vi "Class Object Construction.vi"(6 "class":T1=enum."Valve Controller", 7 "error in":errorcluster, 8 "param2":variant, 9 "param 1":variant, 10 "classes in":T2) -> (0 "error out":errorcluster, 3 "classes out":T2)   [LabVIEW 2011]
uses:
  Controls/Class Objects.ctl
  Modules/File/Configuration/Configuration.lvclass
  Modules/Hardware/Power Supply/Power Supply.lvclass
  Modules/Hardware/Mass Flow Controller/Mass Flow Controller.lvclass
  Modules/Hardware/PID/PID.lvclass
  Modules/Hardware/Valve Controller/Valve Controller.lvclass
  Modules/Hardware/Multimeter/Multimeter.lvclass
  Modules/Hardware/Vapour Generator/Vapour Generator.lvclass
  Modules/File/TDMS/TDMS.lvclass
  Controls/Class Labels.ctl
  Modules/File/Configuration/File Type.ctl
  Controls/TDMS File Handling.ctl
  Functional Global Data/Globals.ctl
  Functional Global Data/Device Params Global.ctl
  Modules/Hardware/INL PID/INL PID.lvclass
  Modules/Hardware/Baseline Mocon piD-Tech plus/Baseline Mocon piD-Tech plus.lvclass
  Modules/Hardware/Stanford Research PS350/Stanford Research PS350.lvclass
  Modules/Hardware/Keithley 2400/Keithley 2400.lvclass
  Modules/Hardware/Owlstone GEN-SYS/Owlstone GEN-SYS.lvclass
  Modules/Hardware/Aalborg GFC17/Aalborg GFC17.lvclass
  Modules/Hardware/INL Valve Controller/INL Valve Controller.lvclass
  Modules/Hardware/Agilent 3458A/Agilent 3458A.lvclass
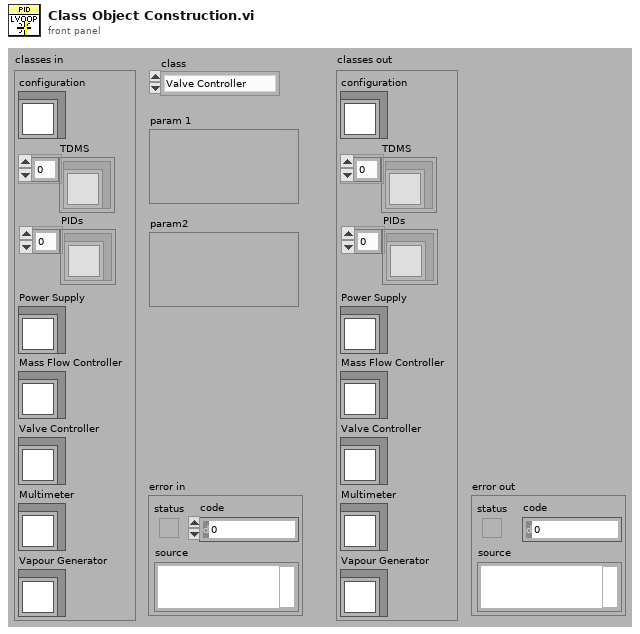
[diagram p1: front panel]
types:
  T1 = typedef "Class Labels.ctl" = enum16{"Configuration", "TDMS", "PID", "Power Supply", "Vapour Generator", "MFC", "NMR", "Valve Controller", "Multimeter"}
  T2 = typedef "Class Objects.ctl" = cluster{"configuration":refnum<class "Configuration.lvclass">, "TDMS":refnum<class "TDMS.lvclass">[], "Power Supply":refnum<class "Power Supply.lvclass">, "Mass Flow Controller":refnum<class "Mass Flow Controller.lvclass">, "Valve Controller":refnum<class "Valve Controller.lvclass">, "Multimeter":refnum<class "Multimeter.lvclass">, "Vapour Generator":refnum<class "Vapour Generator.lvclass">, "PIDs":refnum<class "PID.lvclass">[]}
  T3 = typedef "Configuration.lvclass/File Type.ctl" = enum16{"INI", "XML"}
  T4 = typedef "TDMS File Handling.ctl" = enum16{"Add TDMS File", "Get Active TDMS File", "Set Active TDMS File", "Set Active TDMS File Index"}
  T5 = typedef "Globals.ctl" = enum16{"Initialize", "Get DAQ Params", "Get Data Display Params", "Set DAQ Params", "Set Data Display Params"}
  T6 = typedef "Device Params Global.ctl" = enum16{"Initialize", "Get Device Settings", "Get Device Connections", "Set Device Settings", "Set Device Connections", "Get All Device Properties"}
  T7 = typedef "Data Acquisition Parameters.ctl" = cluster{"Experiment Type":T8, "Experiment Name":string, "Operator Name":string, "Notes":string, "TDMS File Path":path, "Data Acquisition State":bool, "PID Voltage Sweep":T9, "MFC Challenge Profile - Heaviside Step":T10, "MFC Challenge Profile":T11, "MFC Challenge Profile - Staircase":T12}
  T8 = typedef "DAQ Type.ctl" = enum16{"PID Sample", "PID with PS Challenge", "PID with MFC Challenge", "Multimeter Sample", "Multimeter with MFC Challenge"}
  T9 = typedef "PID Voltage Seep Settings.ctl" = cluster{"Voltage Step (V)":dbl, "Voltage Range (V)":cluster{u16, u16}, "Time Step (s)":dbl, "Voltage Step Direction":enum16{"High 2 Low", "Low 2 High"}}
  T10 = typedef "MFC Challenge Profile - Heaviside Step.ctl" = cluster{"Valve Open Duration":u16, "MFC Flow Rate":dbl, "Valve Open Repeats":u16, "Valve Open Start":u16}
  T11 = typedef "MFC Challen Profile Type.ctl" = enum16{"Heaviside", "Staircase"}
  T12 = typedef "MFC Challenge Profile - Staircase.ctl" = cluster{"Step Time Duration":u16, "Step Flow Rate":dbl, "Steps":u16, "Valve Open Start":u16, "Recovery":bool, "Repeats":u16}
  T13 = typedef "Device Connections.ctl" = cluster{"Detector":cluster{"Detector Type":T14, "Connection":bool, "B-M PID":T15, "INL PID Connections":T16}, "Power Supply":cluster{"Type":enum16{"Stanford Research PS350", "Keithley 2400"}, "Connection":bool, "VISA resource name":refnum<visa-resource-name>}, "Mass Flow Controller":cluster{"Type":enum16{"Aalborg GFC17"}, "Connection":bool, "Aalborg GFC17":T18}, "Valve Controller":cluster{"Type":T19, "Connection":bool, "SMC - INL":cluster{"VISA resource name":refnum<visa-resource-name>}}, "Multimeter":cluster{"Multimeter Type":T20, "Connection":bool, "VISA resource name":refnum<visa-resource-name>}, "Vapour Generator":cluster{"Type":T21, "Connection":bool, "Owlstone Gen-SYS":T22}}
  T14 = typedef "Detector Type.ctl" = enum16{"INL PID", "Baseline-Mocon piD-TECH plus"}
  T15 = typedef "Baseline Mocon piD-Tech plus.lvclass/Connections.ctl" = cluster{"AI DAQmx channel":tag}
  T16 = typedef "INL PID Connections.ctl" = cluster{"PIDs":u8, "Integrator DAQ Channels 1":T17, "Integrator DAQ Channels 2":T17}
  T17 = typedef "INL PID.lvclass/Integrator DAQmx Channels.ctl" = cluster{"V0":tag, "S1":tag, "S2":tag}
  T18 = typedef "Aalborg GFC17.lvclass/Aalborg GFC17 Connections.ctl" = cluster{"flow rate setpoint channel":tag, "flow rate reading channel":tag, "valve channel":tag}
  T19 = typedef "Valve Type.ctl" = enum16{"SMC - INL"}
  T20 = typedef "Multimeter Type.ctl" = enum16{"Agilent 3458A"}
  T21 = typedef "Vapour Generator Type.ctl" = enum16{"Owlstone GEN-SYS"}
  T22 = typedef "Owlstone GEN-SYS.lvclass/GEN-SYS Connections.ctl" = cluster{"GEN-SYS VISA resource name":refnum<visa-resource-name>, "OVG-4":cluster{"Flow Address":u8, "Temp Address":u8}, "OHG-4":cluster{"Flow Address":u8, "Easydew VISA resource name":refnum<visa-resource-name>}}
  T23 = enum16{"Stanford Research PS350", "Keithley 2400"}
  T24 = typedef "Device Settings.ctl" = cluster{"PID":cluster{"B-M PID":T25, "INL PID":T26}, "Power Supply":cluster{"Source Value":dbl, "Source Value Units":T27, "Source Mode":T28, "Limits":T29, "Output":bool}, "Mass Flow Controller":cluster{"MFC Flow Rate":dbl, "MFC Valve Status":T32}, "Valve Controller":cluster{"Valve Assembly":T33}, "Multimeter":cluster{"Agilent 3458A":cluster{"Measurement Configuration":T35, "Measurement Integration":T36}}, "Vapour Generator":cluster{"Owlstone Permeation Tube":T37, "Owlstone GEN-SYS Setpoints":T39}}
  T25 = typedef "Baseline Mocon piD-Tech plus.lvclass/Settings.ctl" = cluster{"Detector Sampling Frequency":dbl}
  T26 = typedef "INL PID.lvclass/Settings.ctl" = cluster{"Sampling Frequency":dbl, "Integration Time":dbl, "Integration Periods":u8, "Grid Voltage":dbl}
  T27 = typedef "Power Supply.lvclass/Source Units.ctl" = enum16{"volts", "millivolts", "microvolts", "amps", "milliamps", "microamps", "nanoamps"}
  T28 = typedef "Power Supply.lvclass/Source Mode.ctl" = enum16{"Volts", "Current"}
  T29 = typedef "Power Supply.lvclass/Protection Limits.ctl" = cluster{"Voltage Limit":dbl, "Voltage Limit Units":T30, "Current Limit":dbl, "Current Limit Units":T31, "Voltage Trip/Cmpl":dbl, "Voltage Trip/Cmpl Units":T30, "Current Trip/Cmpl":dbl, "Current Trip/Cmpl Units":T31}
  T30 = typedef "Power Supply.lvclass/Voltage Units.ctl" = enum16{"volts", "millivolts", "microvolts"}
  T31 = typedef "Power Supply.lvclass/Current Units.ctl" = enum16{"amps", "milliamps", "microamps", "nanoamps"}
  T32 = typedef "Mass Flow Controller.lvclass/Valve Status.ctl" = enum16{"Open", "Closed"}
  T33 = typedef "Valve Controller.lvclass/Valve Assembly.ctl" = cluster{"Valve 1":T34, "Valve 2":T34, "Valve 3":T34, "Valve 4":T34, "Valve 5":T34}
  T34 = typedef "Valve Controller.lvclass/Status.ctl" = u16
  T35 = typedef "Agilent 3458A.lvclass/Measurement Configuration.ctl" = cluster{"Function":enum16{"DC Voltage", "AC Voltage", "AC + DC Voltage", "DC Current", "AC Current", "AC + DC Current", "2-Wire Resistance", "4-Wire Resistance", "Frequency", "Period", "Direct Sampling DC", "Direct Sampling AC", "Sub-Sampling DC", "Sub-Sampling AC"}, " Manual Resolution":enum16{"4.5", "5.5", "6.5", "7.5", "8.5"}, "Frequency Source":enum16{"AC + DC Current", "AC + DC Voltage", "AC Current", "AC Voltage"}, "Auto Range":enum16{"OFF", "ON", "ONCE"}}
  T36 = typedef "Agilent 3458A.lvclass/Measurement Integration.ctl" = cluster{"Power Line Cycles":dbl}
  T37 = typedef "Owlstone GEN-SYS.lvclass/Permeation Tube.ctl" = cluster{"Tube":T38, "Molecular Weight":dbl, "Calibration Temperature\n(Celcius)":i32, "Permeation Rate \n(ng/min)":i32}
  T38 = typedef "Owlstone GEN-SYS.lvclass/Permeation Tube Gas.ctl" = enum16{"Isobutylene 27 Nov 2012", "Ammonia 29 Sep 2012", "DMMP Tube A 3 July 2014", "DMMP Tube B 3 July 2014"}
  T39 = typedef "Owlstone GEN-SYS.lvclass/Gen-Sys Setpoints.ctl" = cluster{"OVG-4":cluster{"Oven Temperature":i32, "Sample Flow Rate":i32, "Split Flow Status":u16, "Split Flow Rate":i32}, "OHG-4":cluster{"Wet Air Flow":i32}}
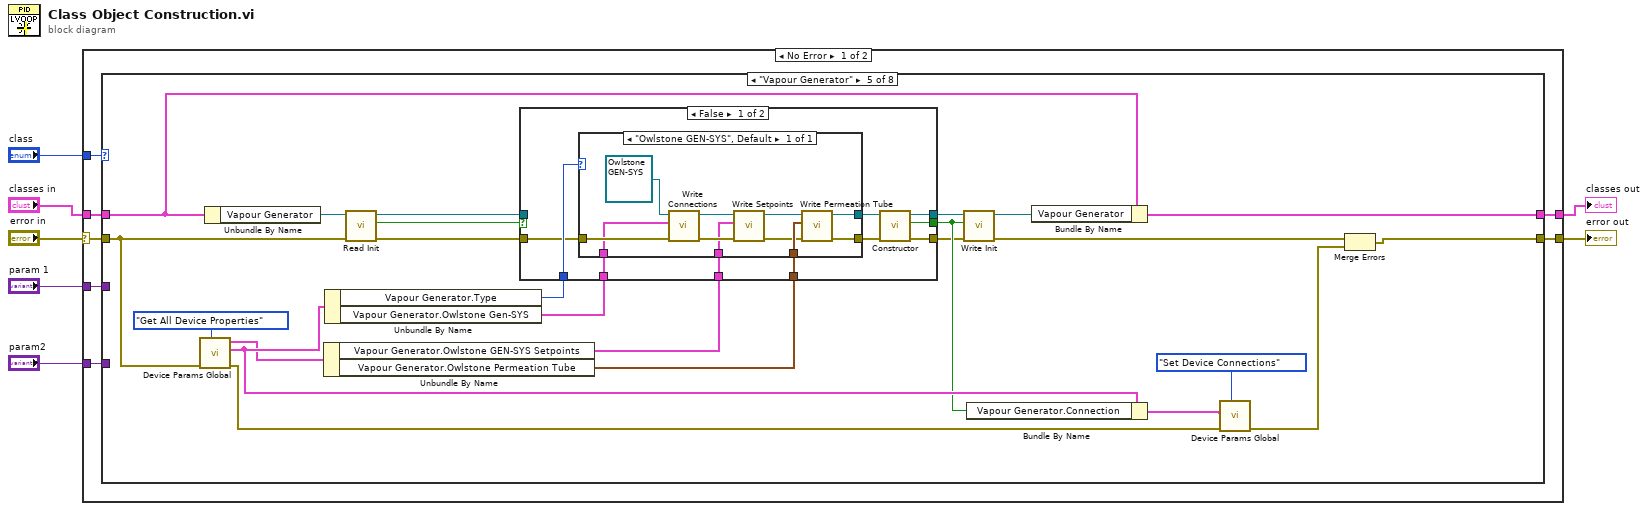
[diagram p0: block diagram]
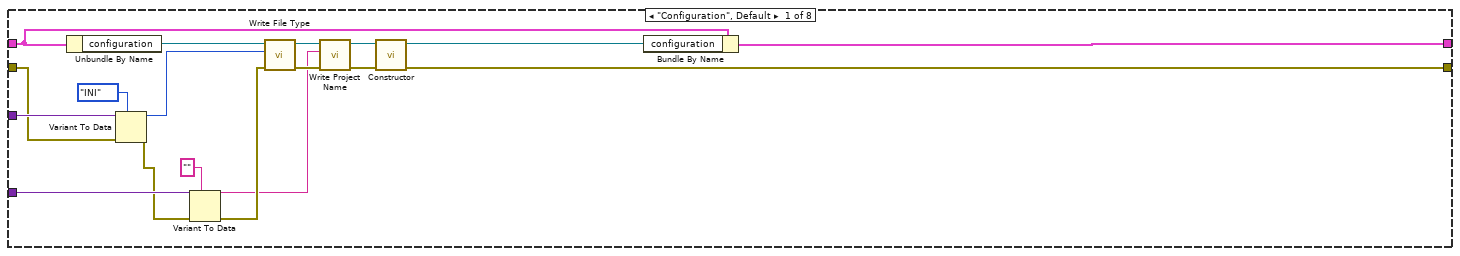
[diagram p2: hidden frame]
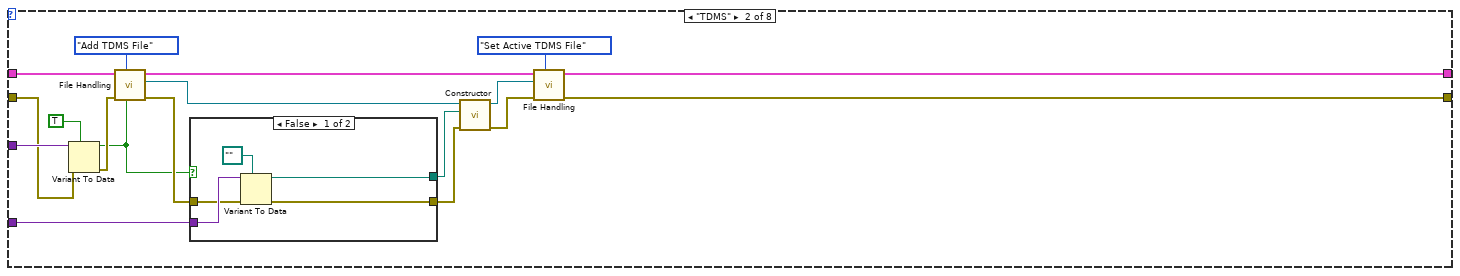
[diagram p3: hidden frame]
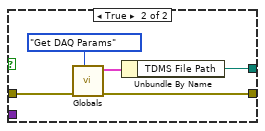
[diagram p4: hidden frame]
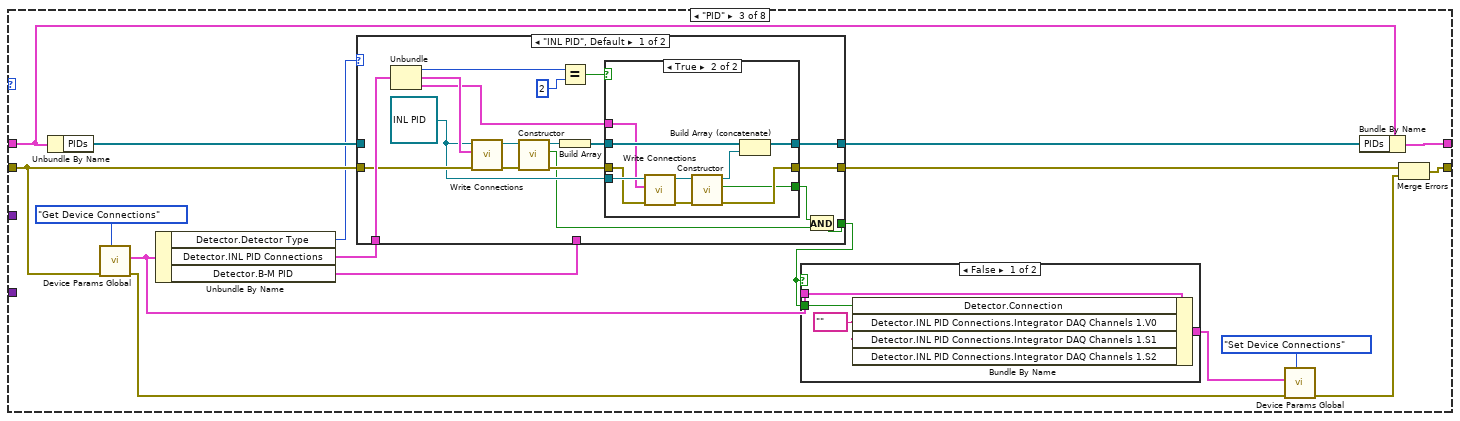
[diagram p5: hidden frame]
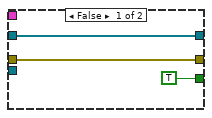
[diagram p6: hidden frame]
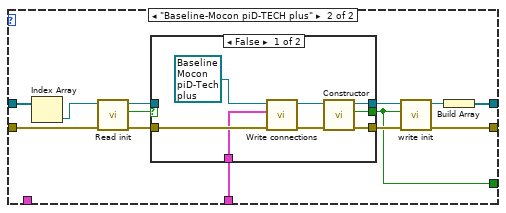
[diagram p7: hidden frame]
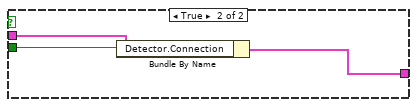
[diagram p9: hidden frame]
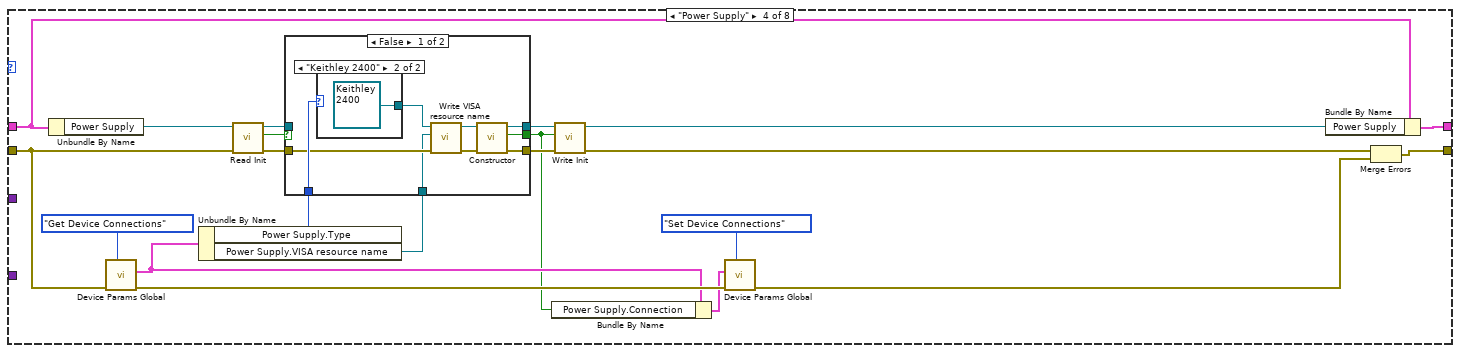
[diagram p10: hidden frame]
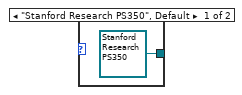
[diagram p11: hidden frame]
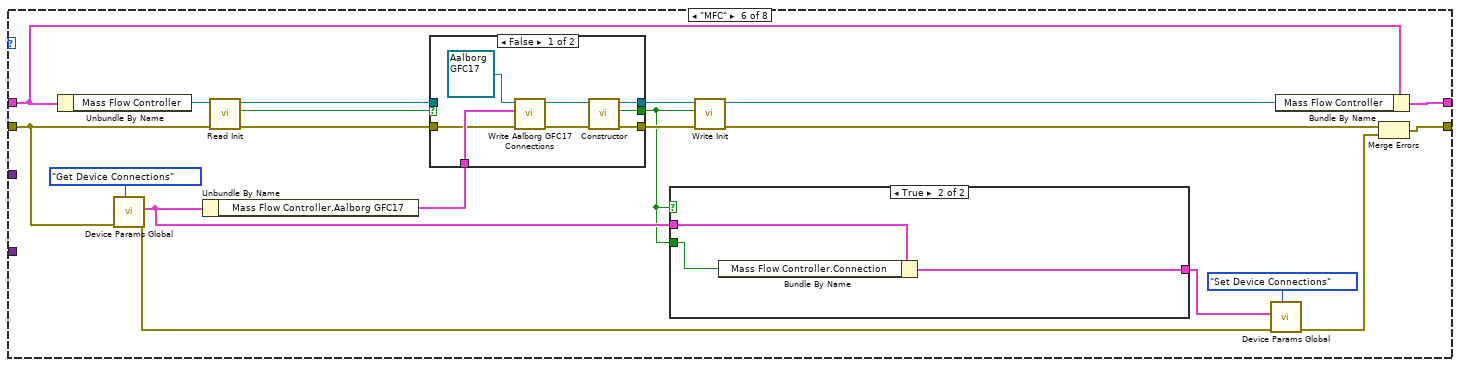
[diagram p14: hidden frame]
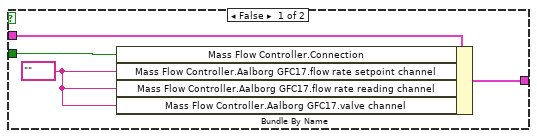
[diagram p15: hidden frame]
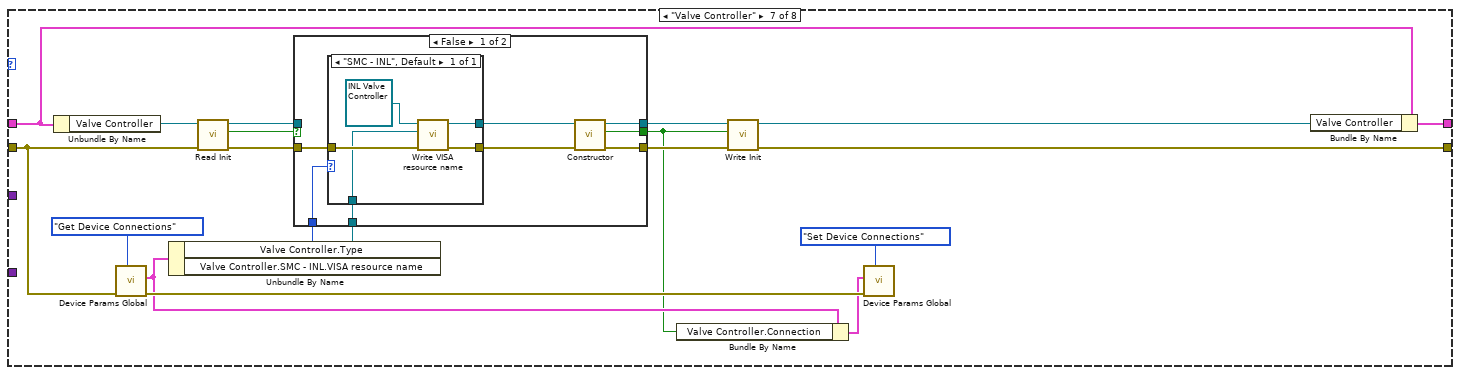
[diagram p17: hidden frame]
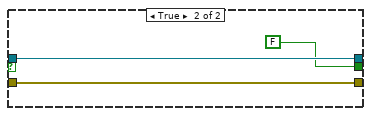
[diagram p18: hidden frame]
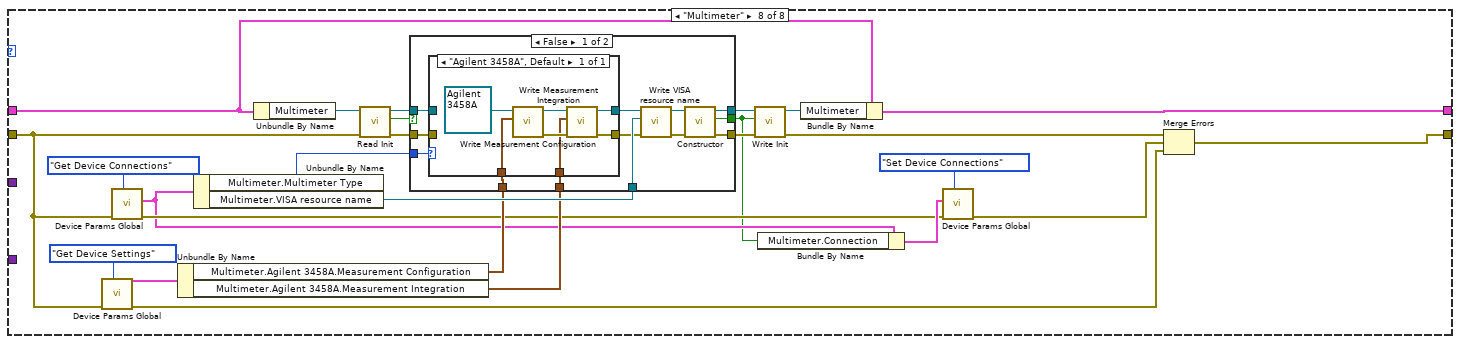
[diagram p19: hidden frame]
diagram:
  n1 = case shown="No Error" "error in" {
    selector: "error in" -> [w8 w346]
    tunnel: [w14 w346] -> w6
    tunnel: "classes in" -> [w13 w345]
    tunnel: "param 1" -> [w12 _]
    tunnel: "param2" -> [w11 _]
    tunnel: "class" -> [w10 _]
    tunnel: [w9 w345] -> w1
    frame No Error {
      n2 = case shown="\"Vapour Generator\"" w10 {
        tunnel: [w30 w43 w75 w154 w180 w229 w266 w310] -> w14
        tunnel: [w32 w44 w77 w156 w198 w237 w278 w320] -> w9
        tunnel: w13 -> [w27 w39 w76 w155 w187 w238 w279 w321]
        tunnel: w12 -> [w29 w40 _ _ _ _ _ _]
        tunnel: w11 -> [w20 w33 _ _ _ _ _ _]
        tunnel: w8 -> [w28 w38 w74 w152 w193 w235 w275 w307]
        frame "Configuration", Default {
          n3 = Unbundle By Name(w27) -> ("configuration"=w26:refnum<class "Configuration.lvclass">)
          n4 = Variant To Data(error in=w28, type=File_Type."INI" ("File Type"), Variant=w29) -> (data=w16:T3, error out=w19:errorcluster)
          n5 = Variant To Data(error in=w19, type="", Variant=w20) -> (data=w15:string, error out=w17:errorcluster)
          n6 = call-dynamic "Write File Type.vi"("error in (no error)"=w17, "File Type"=w16, "Configuration in"=w26) -> ("error out"=w22:errorcluster, "Configuration out"=w25:refnum<class "Configuration.lvclass">)  [unwired: 7 in]
          n7 = call-dynamic "Write Project Name.vi"("error in (no error)"=w22, "Project Name"=w15, "Configuration in"=w25) -> ("error out"=w23:errorcluster, "Configuration out"=w24:refnum<class "Configuration.lvclass">)  [unwired: 7 in]
          n8 = call-dynamic "Constructor.vi"("error in (no error)"=w23, "Configuration in"=w24) -> ("error out"=w30:errorcluster, "Configuration out"=w31:refnum<class "Configuration.lvclass">)  [unwired: 8 in]
          n9 = Bundle By Name(cluster=w27, "configuration"=w31) -> (w32:T2)
        }
        frame "TDMS" {
          n10 = Variant To Data(error in=w38, type=TRUE, Variant=w40) -> (data=w34:bool, error out=w48:errorcluster)
          n11 = call "File Handling.vi"("DAQ?"=w34, "TDMS File Handling"=TDMS_File_Handling."Add TDMS File", "error in"=w48, "Class objects"=w39) -> ("error out"=w37:errorcluster, "TDMS File"=w50:refnum<class "TDMS.lvclass">, "Class objects"=w47:T2)  [unwired: 5 in]
          n12 = case shown="False" w34 {
            tunnel: w37 -> [w53 w58]
            tunnel: [w51 w57] -> w36
            tunnel: [w52 w56] -> w35
            tunnel: w33 -> [w54 _]
            frame False {
              n13 = Variant To Data(error in=w53, type=path "", Variant=w54) -> (data=w52:path, error out=w51:errorcluster)
            }
            frame True {
              n14 = call "Globals.vi"("action"=Globals."Get DAQ Params", "error in"=w58) -> ("error out"=w57:errorcluster, "Data Acquisition"=w60:T7)  [unwired: 7 in, 1 out]
              n15 = Unbundle By Name(w60) -> ("TDMS File Path"=w56:path)
            }
          }
          n16 = call-dynamic "Constructor.vi"("error in"=w36, "path"=w35, "TDMS in"=w50) -> ("error out"=w42:errorcluster, "TDMS out"=w46:refnum<class "TDMS.lvclass">)  [unwired: 7 in]
          n17 = call "File Handling.vi"("TDMS File Handling"=TDMS_File_Handling."Set Active TDMS File", "error in"=w42, "TDMS File"=w46, "Class objects"=w47) -> ("error out"=w43:errorcluster, "Class objects"=w44:T2)  [unwired: 5 in, 1 out]
        }
        frame "PID" {
          n18 = Unbundle By Name(w76) -> ("PIDs"=w64:refnum<class "PID.lvclass">[])
          n19 = call "Device Params Global.vi"("action"=Device_Params_Global."Get Device Connections", "error in"=w74) -> ("error out"=w67:errorcluster, "Device Connections OUT"=w70:T13)  [unwired: 7 in, 1 out]
          n20 = Unbundle By Name(w70) -> ("Detector.Detector Type"=w63:T14, "Detector.INL PID Connections"=w71:T16, "Detector.B-M PID"=w65:T15)
          n21 = case shown="\"INL PID\", Default" w63 {
            tunnel: w74 -> [w92 w118]
            tunnel: [w81 w115] -> w72
            tunnel: w71 -> [w95 _]
            tunnel: w65 -> [_ w114]
            tunnel: w64 -> [_ w110]
            tunnel: [w82 w112] -> w62
            tunnel: [w78 w111] -> w61
            frame "INL PID", Default {
              w85 = refnum<class "INL PID.lvclass"> refnum ("PID.lvclass")
              n22 = Unbundle(w95) -> ("PIDs"=w89:u8, "Integrator DAQ Channels 1"=w94:T17, "Integrator DAQ Channels 2"=w84:T17)
              n23 = call-dynamic "Write Connections.vi"("error in (no error)"=w92, "Integrator DAQ Channels"=w94, "PID in"=w85) -> ("error out"=w91:errorcluster, "PID out"=w93:refnum<class "INL PID.lvclass">)  [unwired: 7 in]
              n24 = call-dynamic "Constructor.vi"("error in"=w91, "PID Detector in"=w93) -> ("error out"=w83:errorcluster, "init"=w80:bool, "PID Detector out"=w90:refnum<class "INL PID.lvclass">)  [unwired: 7 in]
              n25 = Equal?(x=w89, y=u8 2) -> (x = y?=w87:bool)
              n26 = Build Array(w90) -> (w86:refnum<class "INL PID.lvclass">[])
              n27 = case shown="True" w87 {
                tunnel: w86 -> [w98 w105]
                tunnel: w85 -> [_ w106]
                tunnel: w84 -> [_ w103]
                tunnel: w83 -> [w97 w102]
                tunnel: [w98 w101] -> w82
                tunnel: [w97 w100] -> w81
                tunnel: [TRUE ("init") w99] -> w79
                frame False {
                }
                frame True {
                  n28 = call-dynamic "Write Connections.vi"("error in (no error)"=w102, "Integrator DAQ Channels"=w103, "PID in"=w106) -> ("error out"=w107:errorcluster, "PID out"=w108:refnum<class "INL PID.lvclass">)  [unwired: 7 in]
                  n29 = call-dynamic "Constructor.vi"("error in"=w107, "PID Detector in"=w108) -> ("error out"=w100:errorcluster, "init"=w99:bool, "PID Detector out"=w104:refnum<class "INL PID.lvclass">)  [unwired: 7 in]
                  n30 = Build Array (concatenate)(w105, w104) -> (w101:refnum<class "INL PID.lvclass">[])
                }
              }
              n31 = And(x=w79, y=w80) -> (x .and. y?=w78:bool)
            }
            frame "Baseline-Mocon piD-TECH plus" {
              n32 = Index Array(array=w110) -> (element=w109:refnum<class "PID.lvclass">)  [unwired: 1 in]
              n33 = call-dynamic "Read init.vi"("error in (no error)"=w118, "Detector in"=w109) -> ("error out"=w119:errorcluster, "init"=w121:bool, "Detector out"=w120:refnum<class "PID.lvclass">)  [unwired: 7 in]
              n34 = case shown="False" w121 {
                selector: w121 -> [_ w130]
                tunnel: [w129 w132] -> w117
                tunnel: [w128 w131] -> w116
                tunnel: w120 -> [_ w132]
                tunnel: w119 -> [w127 w131]
                tunnel: [w124 w130] -> w111
                tunnel: w114 -> [w123 _]
                frame False {
                  n35 = call-dynamic "Write connections.vi"("error in (no error)"=w127, "Baseline-Mocon piD-TECH plus"=w123, "Baseline Mocon piD-Tech plus in"=refnum<class "Baseline Mocon piD-Tech plus.lvclass"> refnum ("Baseline Mocon piD-Tech plus.lvclass")) -> ("error out"=w125:errorcluster, "Baseline Mocon piD-Tech plus out"=w126:refnum<class "Baseline Mocon piD-Tech plus.lvclass">)  [unwired: 7 in]
                  n36 = call-dynamic "Constructor.vi"("error in"=w125, "Baseline Mocon \npiD-Tech plus in"=w126) -> ("error out"=w128:errorcluster, "init"=w124:bool, "Baseline Mocon \npiD-Tech plus out"=w129:refnum<class "Baseline Mocon piD-Tech plus.lvclass">)  [unwired: 7 in]
                }
                frame True {
                }
              }
              n37 = call-dynamic "write init.vi"("error in (no error)"=w116, "init?"=w111, "Detector in"=w117) -> ("error out"=w115:errorcluster, "Detector out"=w113:refnum<class "PID.lvclass">)  [unwired: 7 in]
              n38 = Build Array(w113) -> (w112:refnum<class "PID.lvclass">[])
            }
          }
          n39 = case shown="False" w61 {
            tunnel: w70 -> [w136 w139]
            tunnel: w61 -> [w135 w138]
            tunnel: [w133 w137] -> w68
            frame False {
              w134 = tag "" ("Detector.PID Connections.Integrator DAQ Channels.V0")
              n40 = Bundle By Name(cluster=w136, "Detector.Connection"=w135, "Detector.INL PID Connections.Integrator DAQ Channels 1.V0"=w134, "Detector.INL PID Connections.Integrator DAQ Channels 1.S1"=w134, "Detector.INL PID Connections.Integrator DAQ Channels 1.S2"=w134) -> (w133:T13)
            }
            frame True {
              n41 = Bundle By Name(cluster=w139, "Detector.Connection"=w138) -> (w137:T13)
            }
          }
          n42 = call "Device Params Global.vi"("action"=Device_Params_Global."Set Device Connections", "error in"=w67, "Device Connections IN"=w68) -> ("error out"=w66:errorcluster)  [unwired: 6 in, 2 out]
          n43 = Bundle By Name(cluster=w76, "PIDs"=w62) -> (w77:T2)
          n44 = Merge Errors(w72, w66) -> (w75:errorcluster)
        }
        frame "Power Supply" {
          n45 = Unbundle By Name(w155) -> ("Power Supply"=w160:refnum<class "Power Supply.lvclass">)
          n46 = call "Device Params Global.vi"("action"=Device_Params_Global."Get Device Connections", "error in"=w152) -> ("error out"=w144:errorcluster, "Device Connections OUT"=w143:T13)  [unwired: 7 in, 1 out]
          n47 = Unbundle By Name(w143) -> ("Power Supply.Type"=w151:T23, "Power Supply.VISA resource name"=w150:refnum<visa-resource-name>)
          n48 = call-dynamic "Read Init.vi"("error in (no error)"=w152, "Power Supply in"=w160) -> ("error out"=w158:errorcluster, "Init"=w159:bool, "Power Supply out"=w157:refnum<class "Power Supply.lvclass">)  [unwired: 7 in]
          n49 = case shown="False" w159 {
            selector: w159 -> [_ w172]
            tunnel: w158 -> [w165 w174]
            tunnel: w157 -> [_ w173]
            tunnel: [w167 w174] -> w147
            tunnel: [w168 w173] -> w149
            tunnel: w151 -> [w169 _]
            tunnel: [w166 w172] -> w142
            tunnel: w150 -> [w162 _]
            frame False {
              n50 = case shown="\"Keithley 2400\"" w169 {
                tunnel: [refnum<class "Stanford Research PS350.lvclass"> refnum ("Stanford Research PS350.lvclass") refnum<class "Keithley 2400.lvclass"> refnum ("Keithley 2400.lvclass")] -> w163
                frame "Stanford Research PS350", Default {
                }
                frame "Keithley 2400" {
                }
              }
              n51 = call-dynamic "Write VISA resource name.vi"("error in (no error)"=w165, "VISA resource name"=w162, "Power Supply in"=w163) -> ("error out"=w164:errorcluster, "Power Supply out"=w161:refnum<class "Power Supply.lvclass">)  [unwired: 7 in]
              n52 = call-dynamic "Constructor.vi"("error in (no error)"=w164, "Power Supply in"=w161) -> ("error out"=w167:errorcluster, "Init"=w166:bool, "Power Supply out"=w168:refnum<class "Power Supply.lvclass">)  [unwired: 7 in]
            }
            frame True {
            }
          }
          n53 = Bundle By Name(cluster=w143, "Power Supply.Connection"=w142) -> (w141:T13)
          n54 = call-dynamic "Write Init.vi"("error in (no error)"=w147, "Init"=w142, "Power Supply in"=w149) -> ("error out"=w146:errorcluster, "Power Supply out"=w148:refnum<class "Power Supply.lvclass">)  [unwired: 7 in]
          n55 = call "Device Params Global.vi"("action"=Device_Params_Global."Set Device Connections", "error in"=w144, "Device Connections IN"=w141) -> ("error out"=w140:errorcluster)  [unwired: 6 in, 2 out]
          n56 = Bundle By Name(cluster=w155, "Power Supply"=w148) -> (w156:T2)
          n57 = Merge Errors(w146, w140) -> (w154:errorcluster)
        }
        frame "Vapour Generator" {
          n58 = call "Device Params Global.vi"("action"=Device_Params_Global."Get All Device Properties", "error in"=w193) -> ("error out"=w176:errorcluster, "Device Connections OUT"=w195:T13, "Device Settings OUT"=w177:T24)  [unwired: 7 in]
          n59 = Unbundle By Name(w187) -> ("Vapour Generator"=w192:refnum<class "Vapour Generator.lvclass">)
          n60 = Unbundle By Name(w177) -> ("Vapour Generator.Owlstone GEN-SYS Setpoints"=w175:T39, "Vapour Generator.Owlstone Permeation Tube"=w178:T37)
          n61 = Unbundle By Name(w195) -> ("Vapour Generator.Type"=w188:T21, "Vapour Generator.Owlstone Gen-SYS"=w179:T22)
          n62 = call-dynamic "Read Init.vi"("error in (no error)"=w193, "Vapour Generator in"=w192) -> ("error out"=w190:errorcluster, "Init"=w191:bool, "Vapour Generator out"=w189:refnum<class "Vapour Generator.lvclass">)  [unwired: 7 in]
          n63 = case shown="False" w191 {
            selector: w191 -> [_ w220]
            tunnel: w190 -> [w207 w221]
            tunnel: w189 -> [_ w222]
            tunnel: w188 -> [w208 _]
            tunnel: [w204 w222] -> w186
            tunnel: [w203 w221] -> w184
            tunnel: [w202 w220] -> w185
            tunnel: w179 -> [w201 _]
            tunnel: w178 -> [w200 _]
            tunnel: w175 -> [w199 _]
            frame False {
              n64 = case shown="\"Owlstone GEN-SYS\", Default" w208 {
                tunnel: w207 -> [w219]
                tunnel: [w215] -> w206
                tunnel: [w216] -> w205
                tunnel: w201 -> [w217]
                tunnel: w200 -> [w214]
                tunnel: w199 -> [w209]
                frame "Owlstone GEN-SYS", Default {
                  n65 = call-dynamic "Write Connections.vi"("error in (no error)"=w219, "Connections"=w217, "Owlstone OVG-4 in"=refnum<class "Owlstone GEN-SYS.lvclass"> refnum ("Owlstone OVG-4.lvclass")) -> ("error out"=w213:errorcluster, "Owlstone OVG-4 out"=w211:refnum<class "Owlstone GEN-SYS.lvclass">)  [unwired: 7 in]
                  n66 = call-dynamic "Write Setpoints.vi"("error in (no error)"=w213, "Setpoints"=w209, "Owlstone GEN-SYS in"=w211) -> ("error out"=w212:errorcluster, "Owlstone GEN-SYS out"=w210:refnum<class "Owlstone GEN-SYS.lvclass">)  [unwired: 7 in]
                  n67 = call-dynamic "Write Permeation Tube.vi"("error in (no error)"=w212, "Permeation Tube"=w214, "Owlstone GEN-SYS in"=w210) -> ("error out"=w216:errorcluster, "Owlstone GEN-SYS out"=w215:refnum<class "Owlstone GEN-SYS.lvclass">)  [unwired: 7 in]
                }
              }
              n68 = call-dynamic "Constructor.vi"("error in"=w205, "Owlstone Gen-SYS in"=w206) -> ("error out"=w203:errorcluster, "Init"=w202:bool, "Owlstone GEN-SYS out"=w204:refnum<class "Owlstone GEN-SYS.lvclass">)  [unwired: 7 in]
            }
            frame True {
            }
          }
          n69 = call-dynamic "Write Init.vi"("error in (no error)"=w184, "Init"=w185, "Vapour Generator in"=w186) -> ("error out"=w182:errorcluster, "Vapour Generator out"=w183:refnum<class "Vapour Generator.lvclass">)  [unwired: 7 in]
          n70 = Bundle By Name(cluster=w195, "Vapour Generator.Connection"=w185) -> (w194:T13)
          n71 = Bundle By Name(cluster=w187, "Vapour Generator"=w183) -> (w198:T2)
          n72 = call "Device Params Global.vi"("action"=Device_Params_Global."Set Device Connections", "error in"=w176, "Device Connections IN"=w194) -> ("error out"=w181:errorcluster)  [unwired: 6 in, 2 out]
          n73 = Merge Errors(w182, w181) -> (w180:errorcluster)
        }
        frame "MFC" {
          n74 = Unbundle By Name(w238) -> ("Mass Flow Controller"=w242:refnum<class "Mass Flow Controller.lvclass">)
          n75 = call "Device Params Global.vi"("action"=Device_Params_Global."Get Device Connections", "error in"=w235) -> ("error out"=w225:errorcluster, "Device Connections OUT"=w228:T13)  [unwired: 7 in, 1 out]
          n76 = Unbundle By Name(w228) -> ("Mass Flow Controller.Aalborg GFC17"=w231:T18)
          n77 = call-dynamic "Read Init.vi"("error in (no error)"=w235, "Mass Flow Controller in"=w242) -> ("error out"=w240:errorcluster, "Init"=w241:bool, "Mass Flow Controller out"=w239:refnum<class "Mass Flow Controller.lvclass">)  [unwired: 7 in]
          n78 = case shown="False" w241 {
            selector: w241 -> [_ w258]
            tunnel: w240 -> [w250 w259]
            tunnel: [w256 w260] -> w233
            tunnel: [w255 w259] -> w234
            tunnel: w239 -> [_ w260]
            tunnel: [w257 w258] -> w227
            tunnel: w231 -> [w252 _]
            frame False {
              n79 = call-dynamic "Write Aalborg GFC17 Connections.vi"("error in (no error)"=w250, "Aalborg GFC17 Connections"=w252, "Aalborg GFC17 in"=refnum<class "Aalborg GFC17.lvclass"> refnum ("Aalborg GFC17.lvclass")) -> ("error out"=w254:errorcluster, "Aalborg GFC17 out"=w253:refnum<class "Aalborg GFC17.lvclass">)  [unwired: 7 in]
              n80 = call-dynamic "Constructor.vi"("error in (no error)"=w254, "Aalborg GFC17 in"=w253) -> ("error out"=w255:errorcluster, "Init"=w257:bool, "Aalborg GFC17 out"=w256:refnum<class "Aalborg GFC17.lvclass">)  [unwired: 7 in]
            }
            frame True {
            }
          }
          n81 = case shown="True" w227 {
            tunnel: w228 -> [w246 w249]
            tunnel: w227 -> [w245 w248]
            tunnel: [w243 w247] -> w226
            frame False {
              w244 = tag "" ("Mass Flow Controller.Aalborg GFC17 Connections.flow rate setpoint channel")
              n82 = Bundle By Name(cluster=w246, "Mass Flow Controller.Connection"=w245, "Mass Flow Controller.Aalborg GFC17.flow rate setpoint channel"=w244, "Mass Flow Controller.Aalborg GFC17.flow rate reading channel"=w244, "Mass Flow Controller.Aalborg GFC17.valve channel"=w244) -> (w243:T13)
            }
            frame True {
              n83 = Bundle By Name(cluster=w249, "Mass Flow Controller.Connection"=w248) -> (w247:T13)
            }
          }
          n84 = call-dynamic "Write Init.vi"("error in (no error)"=w234, "Init"=w227, "Mass Flow Controller in"=w233) -> ("error out"=w230:errorcluster, "Mass Flow Controller out"=w232:refnum<class "Mass Flow Controller.lvclass">)  [unwired: 7 in]
          n85 = call "Device Params Global.vi"("action"=Device_Params_Global."Set Device Connections", "error in"=w225, "Device Connections IN"=w226) -> ("error out"=w223:errorcluster)  [unwired: 6 in, 2 out]
          n86 = Bundle By Name(cluster=w238, "Mass Flow Controller"=w232) -> (w237:T2)
          n87 = Merge Errors(w230, w223) -> (w229:errorcluster)
        }
        frame "Valve Controller" {
          n88 = Unbundle By Name(w279) -> ("Valve Controller"=w276:refnum<class "Valve Controller.lvclass">)
          n89 = call "Device Params Global.vi"("action"=Device_Params_Global."Get Device Connections", "error in"=w275) -> ("error out"=w264:errorcluster, "Device Connections OUT"=w263:T13)  [unwired: 7 in, 1 out]
          n90 = Unbundle By Name(w263) -> ("Valve Controller.Type"=w271:T19, "Valve Controller.SMC - INL.VISA resource name"=w270:refnum<visa-resource-name>)
          n91 = call-dynamic "Read Init.vi"("error in (no error)"=w275, "Valve Controller in"=w276) -> ("error out"=w272:errorcluster, "Init"=w274:bool, "Valve Controller out"=w273:refnum<class "Valve Controller.lvclass">)  [unwired: 7 in]
          n92 = case shown="False" w274 {
            tunnel: [w287 w294] -> w268
            tunnel: [w286 w295] -> w269
            tunnel: w273 -> [_ w295]
            tunnel: w272 -> [w284 w294]
            tunnel: w271 -> [w285 _]
            tunnel: w270 -> [w283 _]
            tunnel: [w280 FALSE ("Init")] -> w262
            frame False {
              n93 = case shown="\"SMC - INL\", Default" w285 {
                tunnel: w284 -> [w292]
                tunnel: w283 -> [w291]
                tunnel: [w289] -> w282
                tunnel: [w288] -> w281
                frame "SMC - INL", Default {
                  n94 = call-dynamic "Write VISA resource name.vi"("error in (no error)"=w292, "VISA resource name"=w291, "INL Valve Controller in"=refnum<class "INL Valve Controller.lvclass"> refnum ("INL Valve Controller.lvclass")) -> ("error out"=w288:errorcluster, "INL Valve Controller out"=w289:refnum<class "INL Valve Controller.lvclass">)  [unwired: 7 in]
                }
              }
              n95 = call-dynamic "Constructor.vi"("error in (no error)"=w281, "INL Valve Controller in"=w282) -> ("error out"=w287:errorcluster, "Init"=w280:bool, "INL Valve Controller out"=w286:refnum<class "INL Valve Controller.lvclass">)  [unwired: 7 in]
            }
            frame True {
            }
          }
          n96 = Bundle By Name(cluster=w263, "Valve Controller.Connection"=w262) -> (w261:T13)
          n97 = call-dynamic "Write Init.vi"("error in (no error)"=w268, "Init"=w262, "Valve Controller in"=w269) -> ("error out"=w266:errorcluster, "Valve Controller out"=w267:refnum<class "Valve Controller.lvclass">)  [unwired: 7 in]
          n98 = call "Device Params Global.vi"("action"=Device_Params_Global."Set Device Connections", "error in"=w264, "Device Connections IN"=w261) -> ()  [unwired: 6 in, 3 out]
          n99 = Bundle By Name(cluster=w279, "Valve Controller"=w267) -> (w278:T2)
        }
        frame "Multimeter" {
          n100 = call "Device Params Global.vi"("action"=Device_Params_Global."Get Device Settings", "error in"=w307) -> ("error out"=w303:errorcluster, "Device Settings OUT"=w305:T24)  [unwired: 7 in, 1 out]
          n101 = call "Device Params Global.vi"("action"=Device_Params_Global."Get Device Connections", "error in"=w307) -> ("error out"=w299:errorcluster, "Device Connections OUT"=w298:T13)  [unwired: 7 in, 1 out]
          n102 = Unbundle By Name(w305) -> ("Multimeter.Agilent 3458A.Measurement Configuration"=w304:T35, "Multimeter.Agilent 3458A.Measurement Integration"=w302:T36)
          n103 = Unbundle By Name(w298) -> ("Multimeter.Multimeter Type"=w308:T20, "Multimeter.VISA resource name"=w309:refnum<visa-resource-name>)
          n104 = Unbundle By Name(w321) -> ("Multimeter"=w319:refnum<class "Multimeter.lvclass">)
          n105 = call-dynamic "Read Init.vi"("error in (no error)"=w307, "Multimeter in"=w319) -> ("error out"=w317:errorcluster, "Init"=w316:bool, "Multimeter out"=w318:refnum<class "Multimeter.lvclass">)  [unwired: 7 in]
          n106 = case shown="False" w316 {
            selector: w316 -> [_ w342]
            tunnel: [w334 w344] -> w315
            tunnel: [w333 w343] -> w314
            tunnel: w318 -> [w327 w344]
            tunnel: w317 -> [w325 w343]
            tunnel: [w332 w342] -> w297
            tunnel: w309 -> [w329 _]
            tunnel: w308 -> [w328 _]
            tunnel: w304 -> [w326 _]
            tunnel: w302 -> [w322 _]
            frame False {
              n107 = case shown="\"Agilent 3458A\", Default" w328 {
                tunnel: w327 -> [_]
                tunnel: w326 -> [w341]
                tunnel: w325 -> [_]
                tunnel: [w335] -> w324
                tunnel: [w336] -> w323
                tunnel: w322 -> [w337]
                frame "Agilent 3458A", Default {
                  n108 = call-dynamic "Write Measurement Configuration.vi"("Measurement Configuration"=w341, "Agilent 3458A in"=refnum<class "Agilent 3458A.lvclass"> refnum ("Agilent 3458A.lvclass")) -> ("error out"=w338:errorcluster, "Agilent 3458A out"=w339:refnum<class "Agilent 3458A.lvclass">)  [unwired: 8 in]
                  n109 = call-dynamic "Write Measurement Integration.vi"("error in (no error)"=w338, "Measurement Integration"=w337, "Agilent 3458A in"=w339) -> ("error out"=w336:errorcluster, "Agilent 3458A out"=w335:refnum<class "Agilent 3458A.lvclass">)  [unwired: 7 in]
                }
              }
              n110 = call-dynamic "Write VISA resource name.vi"("error in (no error)"=w323, "VISA resource name"=w329, "Multimeter in"=w324) -> ("error out"=w331:errorcluster, "Multimeter out"=w330:refnum<class "Agilent 3458A.lvclass">)  [unwired: 7 in]
              n111 = call-dynamic "Constructor.vi"("error in (no error)"=w331, "Agilent 3458A in"=w330) -> ("error out"=w333:errorcluster, "Init"=w332:bool, "Agilent 3458A out"=w334:refnum<class "Agilent 3458A.lvclass">)  [unwired: 7 in]
            }
            frame True {
            }
          }
          n112 = call-dynamic "Write Init.vi"("error in (no error)"=w314, "Init"=w297, "Multimeter in"=w315) -> ("error out"=w311:errorcluster, "Multimeter out"=w313:refnum<class "Multimeter.lvclass">)  [unwired: 7 in]
          n113 = Bundle By Name(cluster=w298, "Multimeter.Connection"=w297) -> (w300:T13)
          n114 = Bundle By Name(cluster=w321, "Multimeter"=w313) -> (w320:T2)
          n115 = call "Device Params Global.vi"("action"=Device_Params_Global."Set Device Connections", "error in"=w299, "Device Connections IN"=w300) -> ("error out"=w296:errorcluster)  [unwired: 6 in, 2 out]
          n116 = Merge Errors(w311, w296, w303) -> (w310:errorcluster)
        }
      }
    }
    frame Error {
    }
  }
  "error out" <- w6
  "classes out" <- w1
